vi "Transmit.vi"(8 "error in (no error)":errorcluster, 10 "Transfer Group in":refnum<class "Transfer Group.lvclass">, 11 "MockTransceiver in":refnum<class "MockTransceiver.lvclass">) -> (0 "error out":errorcluster, 2 "Transfer Group out":refnum<class "Transfer Group.lvclass">, 3 "MockTransceiver out":refnum<class "MockTransceiver.lvclass">)   [LabVIEW 2017, in "MockTransceiver.lvclass"]
uses:
  MockTransceiver.lvclass
  Engine/Classes/Transfer Group/Transfer Group.lvclass
  MockTransceiver.lvclass/MockTransceiver.ctl
  Engine/Classes/Transceiver/Transceiver.lvclass
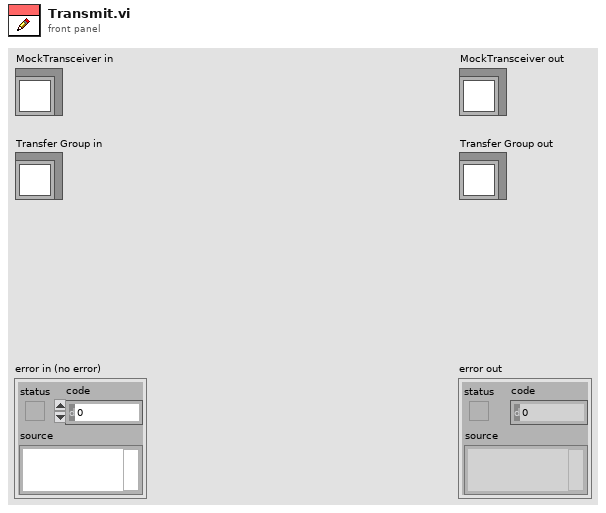
[diagram p1: front panel]
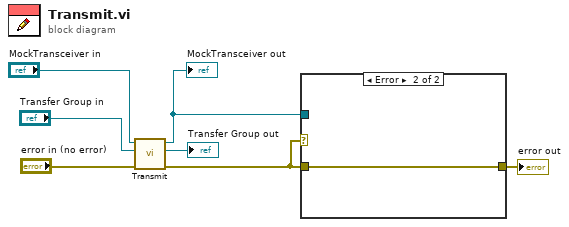
[diagram p0: block diagram]
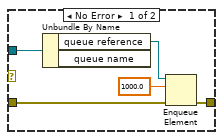
[diagram p2: hidden frame]
diagram:
  n1 = call-parent "Transmit.vi"("error in (no error)"="error in (no error)", "Transfer Group in"="Transfer Group in", "Transceiver in"="MockTransceiver in") -> ("error out"=w1:errorcluster, "Transfer Group out"=→"Transfer Group out":refnum<class "Transfer Group.lvclass">, "Transceiver out"=w3:refnum<class "MockTransceiver.lvclass">)  [unwired: 6 in]
  "MockTransceiver out" <- w3
  n2 = case shown="Error" w1 {
    tunnel: w3 -> [w10 _]
    tunnel: w1 -> [w9 w13]
    tunnel: [w8 w13] -> w2
    frame No Error {
      n3 = Unbundle By Name(w10) -> ("queue reference"=w12:refnum<queue>)  [unwired: 1 out]
      n4 = Enqueue Element(queue=w12, element=1000.0, error in (no error)=w9) -> (error out=w8:errorcluster)  [unwired: 1 in, 2 out]
    }
    frame Error {
    }
  }
  "error out" <- w2
